vi "wrap.GetPaths.vi"(0 "class.GLue in":refnum<class "class.GLue.lvclass">, 11 "error in (no error)":errorcluster) -> (2 "Lpaths":string, 4 "class.GLue out":refnum<class "class.GLue.lvclass">, 13 "Cpaths":string, 15 "error out":errorcluster)   [LabVIEW 2014, in "GLue.lvlib" / "class.GLue.lvclass"]
uses:
  class.GLue.lvclass
  class.GLue.lvclass/class.GLue.ctl
  Resources/GLue.dll
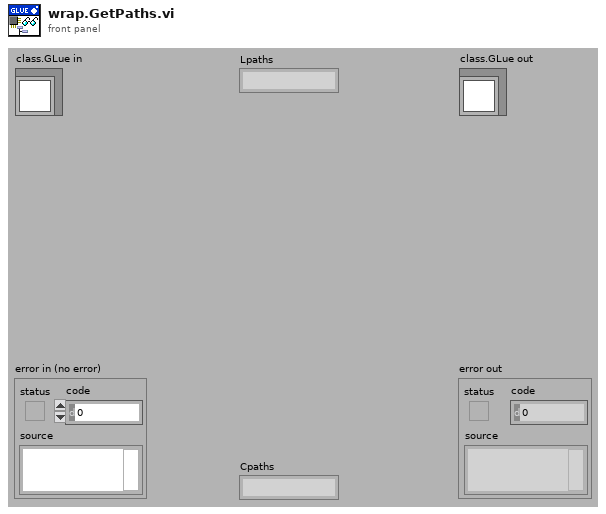
[diagram p1: front panel]
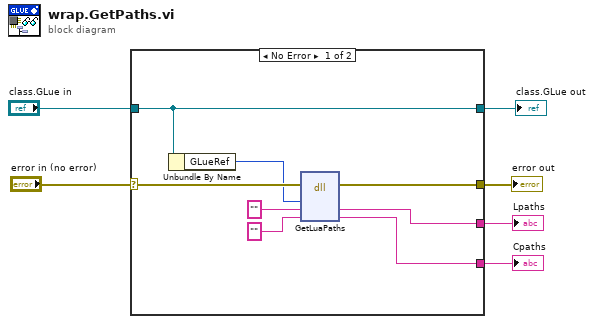
[diagram p0: block diagram]
diagram:
  n1 = case shown="No Error" "error in (no error)" {
    selector: "error in (no error)" -> [w13 w16]
    tunnel: [w12 w16] -> w5
    tunnel: [w14 w15] -> w3
    tunnel: "class.GLue in" -> [w14 w15]
    tunnel: [w8 _] -> w2
    tunnel: [w7 _] -> w1
    frame No Error {
      n2 = Unbundle By Name(w14) -> ("GLueRef"=w11:i64)
      n3 = dll-call lib="C:/Users/Antonie/Documents/work/glue/trunk/Resources/GLue.dll" fn="GetLuaPaths"(error in=w13, "GLue"=w11, "Lpaths"="", "Cpaths"="") -> (error out=w12:errorcluster, "Lpaths"=w8:string, "Cpaths"=w7:string)  [unwired: 4 in, 1 out]
    }
    frame Error {
    }
  }
  "error out" <- w5
  "class.GLue out" <- w3
  "Lpaths" <- w2
  "Cpaths" <- w1
